vi "S4GUI_003.vi"(7 "Tab ObsEng":enum32{"Obs", "CCD modes", "Guider", "Eng"}(tab)) -> ()   [LabVIEW 2018] (continued)
              disable-tunnel: [w4939 w4953] -> w4934
              frame Disabled {
                w4952 = FALSE ("Wait Until Done")
                n2436 = call-dynamic "Read comfile name1.vi"("error in (no error)"=w4941, "Stream in"=w4944) -> ("error out"=w4940:errorcluster, "comfile name1"=w4947:string, "Stream out"=w4942:refnum<class "Stream.lvclass">)  [unwired: 7 in]
                n2437 = call <vilib>:"Application Directory.vi"() -> ("Application Directory"=w4949:path)
                n2438 = Build Path(base path=w4949, name or relative path=w4947) -> (appended path=w4948:path)
                n2439 = Open VI Reference(vi path=w4948, error in (no error)=w4940) -> (vi reference=w4950:refnum<vi>, error out=w4951:errorcluster)  [unwired: 4 in]
                n2440 = invoke class="VI" method="Run VI"(reference=w4950, error in=w4951, "Wait until done"=w4952, "Auto Dispose Ref"=w4952) -> (reference out=w4946:refnum<vi>, error out=w4945:errorcluster)  [unwired: 1 in, 3 out]
                n2441 = call-dynamic "Write commfile ref1.vi"("error in (no error)"=w4945, "commfile ref1"=w4946, "Stream in"=w4942) -> ("error out"=w4939:errorcluster, "Stream out"=w4943:refnum<class "Stream.lvclass">)  [unwired: 7 in]
              }
              frame Enabled {
              }
            }
          }
        }
        n2442 = call-dynamic "Write Stream.vi"("error in (no error)"=w4884, "Stream.lvclass"=w4885, "Server in"=w4886) -> ("error out"=w4894:errorcluster, "Server out"=w4896:refnum<class "Acquisition.lvclass">)  [unwired: 7 in]
        n2443 = call-dynamic "Write enabled.vi"("error in (no error)"=w4894, "enabled"=w4883, "Server in"=w4896) -> ("error out"=w4893:errorcluster, "Server out"=w4895:refnum<class "Acquisition.lvclass">)  [unwired: 7 in]
        n2444 = call-dynamic "Write Channel.vi"("error in (no error)"=w4893, "Channel.lvclass"=w4887, "Acquisition in"=w4895) -> ("error out"=w4901:errorcluster, "Acquisition out"=w4900:refnum<class "Acquisition.lvclass">)  [unwired: 7 in]
        n2445 = call-dynamic "Write AcquisitionD.vi"("error in (no error)"=w4901, "Acquisition.lvclass"=w4900, "S4ACS_GUI in"=w4899) -> ("error out"=w4904:errorcluster, "S4ACS_GUI out"=w4905:refnum<class "S4GUI.lvclass">)  [unwired: 7 in]
      }
      event "Run WPROT": Value Change {
        n2446 = event-data() -> ("NewVal"=w4962:bool)  [unwired: 1 in]
        n2447 = case shown="True" w4962 {
          tunnel: [u32 0 ("Ciclos  WPROT") "Ciclos  WPROT"] -> w4961
          tunnel: w4958 -> [w4964 w4969]
          tunnel: [w4964 w4968] -> w4957
          tunnel: w4956 -> [w4963 w4967]
          tunnel: [w4963 w4966] -> w4955
          frame False {
          }
          frame True {
            n2448 = call-dynamic "Write Obs_state.vi"("error in (no error)"=w4967, "Obs_state"=u32 350, "S4ACS_GUI in"=w4969) -> ("error out"=w4966:errorcluster, "S4ACS_GUI out"=w4968:refnum<class "S4GUI.lvclass">)  [unwired: 7 in]
          }
        }
        n2449 = call-dynamic "Write cycles wprot.vi"("error in (no error)"=w4955, "cycles wprot"=w4961, "S4GUI in"=w4957) -> ("error out"=w4959:errorcluster, "S4GUI out"=w4960:refnum<class "S4GUI.lvclass">)  [unwired: 7 in]
      }
      event "Start SM": Value Change {
        n2450 = event-data() -> ()  [unwired: 1 in, 6 out]
        n2451 = call-dynamic "Read Obs_state.vi"("error in (no error)"=w4998, "S4ACS_GUI in"=w4999) -> ("error out"=w4985:errorcluster, "Obs_state"=w4996:u32, "S4ACS_GUI out"=w4987:refnum<class "S4GUI.lvclass">)  [unwired: 7 in]
        n2452 = call "Read Instrument.lvclass.vi"("error in (no error)"=w4985, "S4ACS_GUI in"=w4987) -> ("error out"=w4983:errorcluster, "Instrument.lvclass"=w4984:refnum<class "Instrument.lvclass">, "S4ACS_GUI out"=w4986:refnum<class "S4GUI.lvclass">)  [unwired: 7 in]
        n2453 = Not Equal?(x=w4996, y=u32 400) -> (x != y?=w4995:bool)
        n2454 = call-dynamic "Read mode.vi"("error in (no error)"=w4983, "Instrument in"=w4984) -> ("error out"=w4982:errorcluster, "mode"=w4981:bool)  [unwired: 7 in, 1 out]
        n2455 = case shown="True" w4995 {
          tunnel: w4986 -> [w5041 w5129]
          tunnel: w4982 -> [w5042 w5128]
          tunnel: [w5045 w5135] -> w4976
          tunnel: [w5044 w5136] -> w4975
          tunnel: w4992 -> [_ w5143]
          tunnel: w4991 -> [_ w5142]
          tunnel: w4990 -> [_ w5141]
          tunnel: w4989 -> [_ w5140]
          tunnel: w4988 -> [_ w5139]
          tunnel: w4981 -> [_ w5138]
          tunnel: w4980 -> [_ w5119]
          tunnel: w4979 -> [_ w5122]
          tunnel: w4978 -> [_ w5121]
          tunnel: w4977 -> [_ w5120]
          tunnel: ["RESUME SM CLICKED" ("User Event") "START SM" ("User Event")] -> w4972
          frame False {
            # "Obs_state=400 (PAUSED), envia RESUME e vai para Obs_state=500 \npara esperar envio do comando RESUME a todos os canais."
            n2456 = call-dynamic "Write Obs_state.vi"("error in (no error)"=w5042, "Obs_state"=500, "S4ACS_GUI in"=w5041) -> ("error out"=w5046:errorcluster, "S4ACS_GUI out"=w5047:refnum<class "S4GUI.lvclass">)  [unwired: 7 in]
            n2457 = call-dynamic "Read AcquisitionA.vi"("error in (no error)"=w5046, "S4ACS_GUI in"=w5047) -> ("error out"=w5033:errorcluster, "Acquisition.lvclass"=w5037:refnum<class "Acquisition.lvclass">, "S4ACS_GUI out"=w5057:refnum<class "S4GUI.lvclass">)  [unwired: 7 in]
            n2458 = call-dynamic "Read enabled.vi"("error in (no error)"=w5033, "Server in"=w5037) -> ("error out"=w5035:errorcluster, "enabled"=w5034:bool, "Server out"=w5036:refnum<class "Acquisition.lvclass">)  [unwired: 7 in]
            n2459 = call-dynamic "Read Channel.vi"("error in (no error)"=w5035, "Acquisition in"=w5036) -> ("error out"=w5038:errorcluster, "Channel.lvclass"=w5039:refnum<class "Channel.lvclass">, "Acquisition out"=w5056:refnum<class "Acquisition.lvclass">)  [unwired: 7 in]
            n2460 = case shown="True" w5034 {
              tunnel: w5056 -> [w5104 w5117]
              tunnel: [w5104 w5116] -> w5055
              tunnel: [w5103 w5113] -> w5054
              tunnel: w5039 -> [_ w5106]
              tunnel: w5038 -> [w5103 w5105]
              frame False {
              }
              frame True {
                n2461 = call-dynamic "Read State Machine.vi"("error in (no error)"=w5105, "Device in"=w5106) -> ("error out"=w5107:errorcluster, "State Machine.lvclass"=w5108:refnum<class "State Machine.lvclass">, "Device out"=w5112:refnum<class "Channel.lvclass">)  [unwired: 7 in]
                n2462 = call "Next State.vi"("error in (no error)"=w5107, "New_State"=96, "State Machine in"=w5108) -> ("error out"=w5109:errorcluster, "State Machine out"=w5111:refnum<class "State Machine.lvclass">)  [unwired: 7 in]
                n2463 = call-dynamic "Write State Machine.vi"("error in (no error)"=w5109, "State Machine.lvclass"=w5111, "Device in"=w5112) -> ("error out"=w5114:errorcluster, "Device out"=w5115:refnum<class "Channel.lvclass">)  [unwired: 7 in]
                n2464 = call-dynamic "Write Channel.vi"("error in (no error)"=w5114, "Channel.lvclass"=w5115, "Acquisition in"=w5117) -> ("error out"=w5113:errorcluster, "Acquisition out"=w5116:refnum<class "Acquisition.lvclass">)  [unwired: 7 in]
              }
            }
            n2465 = call-dynamic "Write AcquisitionA.vi"("error in (no error)"=w5054, "Acquisition.lvclass"=w5055, "S4ACS_GUI in"=w5057) -> ("error out"=w5053:errorcluster, "S4ACS_GUI out"=w5050:refnum<class "S4GUI.lvclass">)  [unwired: 7 in]
            n2466 = call "Read AcquisitionB.vi"("error in (no error)"=w5053, "S4ACS_GUI in"=w5050) -> ("error out"=w5024:errorcluster, "Acquisition.lvclass"=w5025:refnum<class "Acquisition.lvclass">, "S4ACS_GUI out"=w5026:refnum<class "S4GUI.lvclass">)  [unwired: 7 in]
            n2467 = call-dynamic "Read enabled.vi"("error in (no error)"=w5024, "Server in"=w5025) -> ("error out"=w5028:errorcluster, "enabled"=w5027:bool, "Server out"=w5029:refnum<class "Acquisition.lvclass">)  [unwired: 7 in]
            n2468 = call-dynamic "Read Channel.vi"("error in (no error)"=w5028, "Acquisition in"=w5029) -> ("error out"=w5030:errorcluster, "Channel.lvclass"=w5031:refnum<class "Channel.lvclass">, "Acquisition out"=w5032:refnum<class "Acquisition.lvclass">)  [unwired: 7 in]
            n2469 = case shown="True" w5027 {
              tunnel: w5032 -> [w5089 w5102]
              tunnel: [w5089 w5101] -> w5023
              tunnel: [w5088 w5098] -> w5022
              tunnel: w5031 -> [_ w5091]
              tunnel: w5030 -> [w5088 w5090]
              frame False {
              }
              frame True {
                n2470 = call-dynamic "Read State Machine.vi"("error in (no error)"=w5090, "Device in"=w5091) -> ("error out"=w5092:errorcluster, "State Machine.lvclass"=w5093:refnum<class "State Machine.lvclass">, "Device out"=w5097:refnum<class "Channel.lvclass">)  [unwired: 7 in]
                n2471 = call "Next State.vi"("error in (no error)"=w5092, "New_State"=96, "State Machine in"=w5093) -> ("error out"=w5094:errorcluster, "State Machine out"=w5096:refnum<class "State Machine.lvclass">)  [unwired: 7 in]
                n2472 = call-dynamic "Write State Machine.vi"("error in (no error)"=w5094, "State Machine.lvclass"=w5096, "Device in"=w5097) -> ("error out"=w5099:errorcluster, "Device out"=w5100:refnum<class "Channel.lvclass">)  [unwired: 7 in]
                n2473 = call-dynamic "Write Channel.vi"("error in (no error)"=w5099, "Channel.lvclass"=w5100, "Acquisition in"=w5102) -> ("error out"=w5098:errorcluster, "Acquisition out"=w5101:refnum<class "Acquisition.lvclass">)  [unwired: 7 in]
              }
            }
            n2474 = call "Write AcquisitionB.vi"("error in (no error)"=w5022, "Acquisition.lvclass"=w5023, "S4ACS_GUI in"=w5026) -> ("error out"=w5052:errorcluster, "S4ACS_GUI out"=w5049:refnum<class "S4GUI.lvclass">)  [unwired: 7 in]
            n2475 = call-dynamic "Read AcquisitionC.vi"("error in (no error)"=w5052, "S4ACS_GUI in"=w5049) -> ("error out"=w5012:errorcluster, "Acquisition.lvclass"=w5015:refnum<class "Acquisition.lvclass">, "S4ACS_GUI out"=w5014:refnum<class "S4GUI.lvclass">)  [unwired: 7 in]
            n2476 = call-dynamic "Read enabled.vi"("error in (no error)"=w5012, "Server in"=w5015) -> ("error out"=w5017:errorcluster, "enabled"=w5016:bool, "Server out"=w5018:refnum<class "Acquisition.lvclass">)  [unwired: 7 in]
            n2477 = call-dynamic "Read Channel.vi"("error in (no error)"=w5017, "Acquisition in"=w5018) -> ("error out"=w5019:errorcluster, "Channel.lvclass"=w5020:refnum<class "Channel.lvclass">, "Acquisition out"=w5021:refnum<class "Acquisition.lvclass">)  [unwired: 7 in]
            n2478 = case shown="True" w5016 {
              tunnel: w5021 -> [w5074 w5087]
              tunnel: [w5074 w5086] -> w5013
              tunnel: [w5073 w5083] -> w5011
              tunnel: w5020 -> [_ w5076]
              tunnel: w5019 -> [w5073 w5075]
              frame False {
              }
              frame True {
                n2479 = call-dynamic "Read State Machine.vi"("error in (no error)"=w5075, "Device in"=w5076) -> ("error out"=w5077:errorcluster, "State Machine.lvclass"=w5078:refnum<class "State Machine.lvclass">, "Device out"=w5082:refnum<class "Channel.lvclass">)  [unwired: 7 in]
                n2480 = call "Next State.vi"("error in (no error)"=w5077, "New_State"=96, "State Machine in"=w5078) -> ("error out"=w5079:errorcluster, "State Machine out"=w5081:refnum<class "State Machine.lvclass">)  [unwired: 7 in]
                n2481 = call-dynamic "Write State Machine.vi"("error in (no error)"=w5079, "State Machine.lvclass"=w5081, "Device in"=w5082) -> ("error out"=w5084:errorcluster, "Device out"=w5085:refnum<class "Channel.lvclass">)  [unwired: 7 in]
                n2482 = call-dynamic "Write Channel.vi"("error in (no error)"=w5084, "Channel.lvclass"=w5085, "Acquisition in"=w5087) -> ("error out"=w5083:errorcluster, "Acquisition out"=w5086:refnum<class "Acquisition.lvclass">)  [unwired: 7 in]
              }
            }
            n2483 = call-dynamic "Write AcquisitionC.vi"("error in (no error)"=w5011, "Acquisition.lvclass"=w5013, "S4ACS_GUI in"=w5014) -> ("error out"=w5051:errorcluster, "S4ACS_GUI out"=w5048:refnum<class "S4GUI.lvclass">)  [unwired: 7 in]
            n2484 = call-dynamic "Read AcquisitionD.vi"("error in (no error)"=w5051, "S4ACS_GUI in"=w5048) -> ("error out"=w5002:errorcluster, "Acquisition.lvclass"=w5003:refnum<class "Acquisition.lvclass">, "S4ACS_GUI out"=w5004:refnum<class "S4GUI.lvclass">)  [unwired: 7 in]
            n2485 = call-dynamic "Read enabled.vi"("error in (no error)"=w5002, "Server in"=w5003) -> ("error out"=w5006:errorcluster, "enabled"=w5005:bool, "Server out"=w5007:refnum<class "Acquisition.lvclass">)  [unwired: 7 in]
            n2486 = call-dynamic "Read Channel.vi"("error in (no error)"=w5006, "Acquisition in"=w5007) -> ("error out"=w5008:errorcluster, "Channel.lvclass"=w5009:refnum<class "Channel.lvclass">, "Acquisition out"=w5010:refnum<class "Acquisition.lvclass">)  [unwired: 7 in]
            n2487 = case shown="True" w5005 {
              tunnel: w5010 -> [w5059 w5072]
              tunnel: [w5059 w5071] -> w5001
              tunnel: [w5058 w5068] -> w5000
              tunnel: w5009 -> [_ w5061]
              tunnel: w5008 -> [w5058 w5060]
              frame False {
              }
              frame True {
                n2488 = call-dynamic "Read State Machine.vi"("error in (no error)"=w5060, "Device in"=w5061) -> ("error out"=w5062:errorcluster, "State Machine.lvclass"=w5063:refnum<class "State Machine.lvclass">, "Device out"=w5067:refnum<class "Channel.lvclass">)  [unwired: 7 in]
                n2489 = call "Next State.vi"("error in (no error)"=w5062, "New_State"=96, "State Machine in"=w5063) -> ("error out"=w5064:errorcluster, "State Machine out"=w5066:refnum<class "State Machine.lvclass">)  [unwired: 7 in]
                n2490 = call-dynamic "Write State Machine.vi"("error in (no error)"=w5064, "State Machine.lvclass"=w5066, "Device in"=w5067) -> ("error out"=w5069:errorcluster, "Device out"=w5070:refnum<class "Channel.lvclass">)  [unwired: 7 in]
                n2491 = call-dynamic "Write Channel.vi"("error in (no error)"=w5069, "Channel.lvclass"=w5070, "Acquisition in"=w5072) -> ("error out"=w5068:errorcluster, "Acquisition out"=w5071:refnum<class "Acquisition.lvclass">)  [unwired: 7 in]
              }
            }
            n2492 = call-dynamic "Write AcquisitionD.vi"("error in (no error)"=w5000, "Acquisition.lvclass"=w5001, "S4ACS_GUI in"=w5004) -> ("error out"=w5044:errorcluster, "S4ACS_GUI out"=w5045:refnum<class "S4GUI.lvclass">)  [unwired: 7 in]
          }
          frame True {
            # "vide S4GUI:\nHandleObservationSync.vi"
            # "aba atual em Tab Acq Type"
            n2493 = call "Read Instrument.lvclass.vi"("error in (no error)"=w5128, "S4ACS_GUI in"=w5129) -> ("error out"=w5131:errorcluster, "Instrument.lvclass"=w5133:refnum<class "Instrument.lvclass">, "S4ACS_GUI out"=w5126:refnum<class "S4GUI.lvclass">)  [unwired: 7 in]
            n2494 = call "Read WPROT.vi"("error in (no error)"=w5131, "Instrument in"=w5133) -> ("error out"=w5130:errorcluster, "Opt_Selector.lvclass"=w5132:refnum<class "Opt_Selector.lvclass">)  [unwired: 7 in, 1 out]
            n2495 = call-dynamic "Read sequencia.vi"("error in (no error)"=w5130, "Opt_Selector in"=w5132) -> ("error out"=w5125:errorcluster, "sequencia"=w5127:u16)  [unwired: 7 in, 1 out]
            n2496 = case shown="\"FOCUS\"" w5119 {
              tunnel: [u32 271 ("Obs_state") u32 251 ("Obs_state")] -> w5146
              tunnel: w5126 -> [w5167 w5170]
              tunnel: w5125 -> [w5157 w5169]
              tunnel: [w5165 w5170] -> w5124
              tunnel: [w5156 w5169] -> w5123
              tunnel: w5122 -> [w5164 _]
              tunnel: w5121 -> [w5163 _]
              tunnel: w5120 -> [w5162 _]
              frame "FOCUS" {
                n2497 = call-dynamic "Read TelFocus.lvclass.vi"("error in (no error)"=w5157, "S4GUI in"=w5167) -> ("error out"=w5159:errorcluster, "TelFocus.lvclass"=w5161:refnum<class "TelFocus.lvclass">, "S4GUI out"=w5166:refnum<class "S4GUI.lvclass">)  [unwired: 7 in]
                n2498 = call-dynamic "LoadParam.vi"("#steps"=w5162, "error in (no error)"=w5159, "step"=w5163, "init"=w5164, "TelFocus in"=w5161) -> ("error out"=w5158:errorcluster, "TelFocus out"=w5160:refnum<class "TelFocus.lvclass">)  [unwired: 5 in]
                n2499 = call-dynamic "Write TelFocus.lvclass.vi"("error in (no error)"=w5158, "TelFocus.lvclass"=w5160, "S4GUI in"=w5166) -> ("error out"=w5156:errorcluster, "S4GUI out"=w5165:refnum<class "S4GUI.lvclass">)  [unwired: 7 in]
              }
              frame Default {
              }
            }
            n2500 = case shown="\"FOCUS\"" w5119 {
              tunnel: w5138 -> [_ w5152]
              tunnel: [u32 1 ("# Cycles") w5151] -> w5137
              tunnel: [u32 1 w5150] -> w5134
              tunnel: w5127 -> [_ w5149]
              frame "FOCUS" {
                # "Aba FOCUS: Para a sequencia de foco, sempre  #Cycles=1 e #Seqs=1"
              }
              frame Default {
                n2501 = case shown="False" w5152 {
                  tunnel: [0 w5155] -> w5150
                  tunnel: w5149 -> [_ w5154]
                  frame False {
                    # "OV 20230424: \n#SEQ agora armazena as\nposições da lâmina utilizadas.\nNa fotometria, #SEQ=0"
                    # "fotometria:"
                  }
                  frame True {
                    # "OV 20230424: \n#SEQ agora armazena as\nposições da lâmina utilizadas.\nNa polarimetria, #SEQ=WPROT.sequencia"
                    # "polarimetria:"
                    n2502 = To Unsigned Long Integer(number=w5154) -> (unsigned 32bit integer=w5155:u32)
                  }
                }
                n2503 = local read "# Cycles"() -> (w5151:u32)
              }
            }
            n2504 = call-dynamic "Write Obs_state.vi"("error in (no error)"=w5123, "Obs_state"=w5146, "S4ACS_GUI in"=w5124) -> ("error out"=w5145:errorcluster, "S4ACS_GUI out"=w5144:refnum<class "S4GUI.lvclass">)  [unwired: 7 in]
            n2505 = stacked-sequence {
              seq-local: [w5194 _ _ _] -> [_ w5266 _ _]
              seq-local: [w5193 _ _ _] -> [_ w5265 _ _]
              seq-local: [_ w5264 _ _] -> [_ _ w5317 _]
              seq-local: [_ w5263 _ _] -> [_ _ w5316 _]
              seq-local: [_ _ w5315 _] -> [_ _ _ w5368]
              seq-local: [_ _ w5314 _] -> [_ _ _ w5367]
              tunnel: w5145 -> [w5209 _ _ _]
              tunnel: w5144 -> [w5208 _ _ _]
              tunnel: [_ _ _ w5366] -> w5135
              tunnel: [_ _ _ w5365] -> w5136
              tunnel: w5143 -> [w5192 w5262 w5313 w5364]
              tunnel: w5142 -> [w5191 w5261 w5293 w5344]
              tunnel: w5141 -> [w5190 w5241 w5292 w5343]
              tunnel: w5140 -> [w5189 w5240 w5291 w5342]
              tunnel: w5139 -> [w5184 w5237 w5288 w5339]
              tunnel: w5137 -> [_ _ _ _]
              tunnel: w5134 -> [_ _ _ _]
              tunnel: w5119 -> [w5176 w5231 w5282 w5331]
              frame #0 {
                # "object"
                # "suffix"
                # "obsType"
                n2506 = local read "Exptime ch1"() -> (w5177:dbl)
                n2507 = call-dynamic "Read AcquisitionA.vi"("error in (no error)"=w5209, "S4ACS_GUI in"=w5208) -> ("error out"=w5207:errorcluster, "Acquisition.lvclass"=w5206:refnum<class "Acquisition.lvclass">, "S4ACS_GUI out"=w5197:refnum<class "S4GUI.lvclass">)  [unwired: 7 in]
                n2508 = call-dynamic "Read Channel.vi"("error in (no error)"=w5207, "Acquisition in"=w5206) -> ("error out"=w5204:errorcluster, "Channel.lvclass"=w5205:refnum<class "Channel.lvclass">, "Acquisition out"=w5196:refnum<class "Acquisition.lvclass">)  [unwired: 7 in]
                n2509 = call-dynamic "Read Interface.vi"("error in (no error)"=w5204, "Channel in"=w5205) -> ("error out"=w5215:errorcluster, "Interface.lvclass"=w5202:refnum<class "Interface.lvclass">, "Channel out"=w5203:refnum<class "Channel.lvclass">)  [unwired: 7 in]
                n2510 = call "Write Exposure Time.vi"("error in (no error)"=w5215, "Exposure Time"=w5177, "Interface in"=w5202) -> ("error out"=w5178:errorcluster, "Interface out"=w5181:refnum<class "Interface.lvclass">)  [unwired: 7 in]
                n2511 = case shown="Default" w5176 {
                  tunnel: w5181 -> [w5217 w5222]
                  tunnel: [w5217 w5221] -> w5180
                  tunnel: [w5216 w5220] -> w5179
                  tunnel: w5178 -> [w5216 w5219]
                  tunnel: w5177 -> [_ w5218]
                  frame "ZERO" {
                  }
                  frame Default {
                    n2512 = call-dynamic "Write prev ExpTime.vi"("error in (no error)"=w5219, "prev ExpTime"=w5218, "Interface in"=w5222) -> ("error out"=w5220:errorcluster, "Interface out"=w5221:refnum<class "Interface.lvclass">)  [unwired: 7 in]
                  }
                }
                n2513 = call-dynamic "Write Suffix.vi"("error in (no error)"=w5179, "Suffix"=w5192, "Interface in"=w5180) -> ("error out"=w5214:errorcluster, "Interface out"=w5201:refnum<class "Interface.lvclass">)  [unwired: 7 in]
                n2514 = call-dynamic "Write ObsType.vi"("error in (no error)"=w5214, "ObsType"=w5190, "Interface in"=w5201) -> ("error out"=w5213:errorcluster, "Interface out"=w5200:refnum<class "Interface.lvclass">)  [unwired: 7 in]
                n2515 = call-dynamic "Write Object.vi"("error in (no error)"=w5213, "Object"=w5189, "Interface in"=w5200) -> ("error out"=w5212:errorcluster, "Interface out"=w5199:refnum<class "Interface.lvclass">)  [unwired: 7 in]
                n2516 = call-dynamic "Write Comments.vi"("error in (no error)"=w5212, "Comments"=w5191, "Interface in"=w5199) -> ("error out"=w5211:errorcluster, "Interface out"=w5198:refnum<class "Interface.lvclass">)  [unwired: 7 in]
                n2517 = call-dynamic "Write DS9.vi"("error in (no error)"=w5211, "DS9"="F", "Interface in"=w5198) -> ("error out"=w5186:errorcluster, "Interface out"=w5188:refnum<class "Interface.lvclass">)  [unwired: 7 in]
                n2518 = call-dynamic "Write Observer.vi"("error in (no error)"=w5186, "Observer"=w5184, "Interface in"=w5188) -> ("error out"=w5185:errorcluster, "Interface out"=w5187:refnum<class "Interface.lvclass">)  [unwired: 7 in]
                n2519 = property on="Exposure Time ch1" class="Slide (strict)"("Scale.Maximum"=w5177, "Scale.Minimum"=0.0 ("Scale.Range:Minimum")) -> ()  [unwired: 2 in, 2 out]
                n2520 = call-dynamic "Write Interface.vi"("error in (no error)"=w5185, "Interface.lvclass"=w5187, "Channel in"=w5203) -> ("error out"=w5183:errorcluster, "Channel out"=w5182:refnum<class "Channel.lvclass">)  [unwired: 7 in]
                n2521 = call-dynamic "Write Channel.vi"("error in (no error)"=w5183, "Channel.lvclass"=w5182, "Acquisition in"=w5196) -> ("error out"=w5173:errorcluster, "Acquisition out"=w5175:refnum<class "Acquisition.lvclass">)  [unwired: 7 in]
                n2522 = call-dynamic "CalcCubeDuration.vi"("error in (no error)"=w5173, "Acquisition in"=w5175) -> ("error out"=w5172:errorcluster, "Acquisition out"=w5174:refnum<class "Acquisition.lvclass">)  [unwired: 8 in]
                n2523 = call-dynamic "Write AcquisitionA.vi"("error in (no error)"=w5172, "Acquisition.lvclass"=w5174, "S4ACS_GUI in"=w5197) -> ("error out"=w5193:errorcluster, "S4ACS_GUI out"=w5194:refnum<class "S4GUI.lvclass">)  [unwired: 7 in]
              }
              frame #1 {
                # "object"
                # "suffix"
                # "obsType"
                n2524 = call "Read AcquisitionB.vi"("error in (no error)"=w5265, "S4ACS_GUI in"=w5266) -> ("error out"=w5249:errorcluster, "Acquisition.lvclass"=w5250:refnum<class "Acquisition.lvclass">, "S4ACS_GUI out"=w5259:refnum<class "S4GUI.lvclass">)  [unwired: 7 in]
                n2525 = local read "Exptime ch2"() -> (w5232:dbl)
                n2526 = call-dynamic "Read Channel.vi"("error in (no error)"=w5249, "Acquisition in"=w5250) -> ("error out"=w5252:errorcluster, "Channel.lvclass"=w5251:refnum<class "Channel.lvclass">, "Acquisition out"=w5260:refnum<class "Acquisition.lvclass">)  [unwired: 7 in]
                n2527 = call-dynamic "Read Interface.vi"("error in (no error)"=w5252, "Channel in"=w5251) -> ("error out"=w5244:errorcluster, "Interface.lvclass"=w5254:refnum<class "Interface.lvclass">, "Channel out"=w5253:refnum<class "Channel.lvclass">)  [unwired: 7 in]
                n2528 = call "Write Exposure Time.vi"("error in (no error)"=w5244, "Exposure Time"=w5232, "Interface in"=w5254) -> ("error out"=w5233:errorcluster, "Interface out"=w5234:refnum<class "Interface.lvclass">)  [unwired: 7 in]
                n2529 = case shown="Default" w5231 {
                  tunnel: w5234 -> [w5268 w5273]
                  tunnel: [w5268 w5272] -> w5230
                  tunnel: [w5267 w5271] -> w5229
                  tunnel: w5233 -> [w5267 w5270]
                  tunnel: w5232 -> [_ w5269]
                  frame "ZERO" {
                  }
                  frame Default {
                    n2530 = call-dynamic "Write prev ExpTime.vi"("error in (no error)"=w5270, "prev ExpTime"=w5269, "Interface in"=w5273) -> ("error out"=w5271:errorcluster, "Interface out"=w5272:refnum<class "Interface.lvclass">)  [unwired: 7 in]
                  }
                }
                n2531 = call-dynamic "Write Suffix.vi"("error in (no error)"=w5229, "Suffix"=w5262, "Interface in"=w5230) -> ("error out"=w5245:errorcluster, "Interface out"=w5255:refnum<class "Interface.lvclass">)  [unwired: 7 in]
                n2532 = call-dynamic "Write ObsType.vi"("error in (no error)"=w5245, "ObsType"=w5241, "Interface in"=w5255) -> ("error out"=w5246:errorcluster, "Interface out"=w5256:refnum<class "Interface.lvclass">)  [unwired: 7 in]
                n2533 = call-dynamic "Write Object.vi"("error in (no error)"=w5246, "Object"=w5240, "Interface in"=w5256) -> ("error out"=w5247:errorcluster, "Interface out"=w5257:refnum<class "Interface.lvclass">)  [unwired: 7 in]
                n2534 = call-dynamic "Write Comments.vi"("error in (no error)"=w5247, "Comments"=w5261, "Interface in"=w5257) -> ("error out"=w5248:errorcluster, "Interface out"=w5258:refnum<class "Interface.lvclass">)  [unwired: 7 in]
                n2535 = call-dynamic "Write DS9.vi"("error in (no error)"=w5248, "DS9"="F", "Interface in"=w5258) -> ("error out"=w5238:errorcluster, "Interface out"=w5239:refnum<class "Interface.lvclass">)  [unwired: 7 in]
                n2536 = call-dynamic "Write Observer.vi"("error in (no error)"=w5238, "Observer"=w5237, "Interface in"=w5239) -> ("error out"=w5223:errorcluster, "Interface out"=w5224:refnum<class "Interface.lvclass">)  [unwired: 7 in]
                n2537 = property on="Exposure Time ch2" class="Slide (strict)"("Scale.Maximum"=w5232, "Scale.Minimum"=0.0 ("Scale.Range:Minimum")) -> ()  [unwired: 2 in, 2 out]
                n2538 = call-dynamic "Write Interface.vi"("error in (no error)"=w5223, "Interface.lvclass"=w5224, "Channel in"=w5253) -> ("error out"=w5236:errorcluster, "Channel out"=w5235:refnum<class "Channel.lvclass">)  [unwired: 7 in]
                n2539 = call-dynamic "Write Channel.vi"("error in (no error)"=w5236, "Channel.lvclass"=w5235, "Acquisition in"=w5260) -> ("error out"=w5226:errorcluster, "Acquisition out"=w5228:refnum<class "Acquisition.lvclass">)  [unwired: 7 in]
                n2540 = call-dynamic "CalcCubeDuration.vi"("error in (no error)"=w5226, "Acquisition in"=w5228) -> ("error out"=w5225:errorcluster, "Acquisition out"=w5227:refnum<class "Acquisition.lvclass">)  [unwired: 8 in]
                n2541 = call "Write AcquisitionB.vi"("error in (no error)"=w5225, "Acquisition.lvclass"=w5227, "S4ACS_GUI in"=w5259) -> ("error out"=w5263:errorcluster, "S4ACS_GUI out"=w5264:refnum<class "S4GUI.lvclass">)  [unwired: 7 in]
              }
              frame #2 {
                # "object"
                # "suffix"
                # "obsType"
                n2542 = call-dynamic "Read AcquisitionC.vi"("error in (no error)"=w5316, "S4ACS_GUI in"=w5317) -> ("error out"=w5307:errorcluster, "Acquisition.lvclass"=w5306:refnum<class "Acquisition.lvclass">, "S4ACS_GUI out"=w5297:refnum<class "S4GUI.lvclass">)  [unwired: 7 in]
                n2543 = call-dynamic "Read Channel.vi"("error in (no error)"=w5307, "Acquisition in"=w5306) -> ("error out"=w5304:errorcluster, "Channel.lvclass"=w5305:refnum<class "Channel.lvclass">, "Acquisition out"=w5296:refnum<class "Acquisition.lvclass">)  [unwired: 7 in]
                n2544 = local read "Exptime ch3"() -> (w5283:dbl)
                n2545 = call-dynamic "Read Interface.vi"("error in (no error)"=w5304, "Channel in"=w5305) -> ("error out"=w5312:errorcluster, "Interface.lvclass"=w5302:refnum<class "Interface.lvclass">, "Channel out"=w5303:refnum<class "Channel.lvclass">)  [unwired: 7 in]
                n2546 = call "Write Exposure Time.vi"("error in (no error)"=w5312, "Exposure Time"=w5283, "Interface in"=w5302) -> ("error out"=w5284:errorcluster, "Interface out"=w5285:refnum<class "Interface.lvclass">)  [unwired: 7 in]
                n2547 = case shown="\"ZERO\"" w5282 {
                  tunnel: w5285 -> [w5319 w5324]
                  tunnel: [w5319 w5323] -> w5281
                  tunnel: [w5318 w5322] -> w5280
                  tunnel: w5284 -> [w5318 w5321]
                  tunnel: w5283 -> [_ w5320]
                  frame "ZERO" {
                  }
                  frame Default {
                    n2548 = call-dynamic "Write prev ExpTime.vi"("error in (no error)"=w5321, "prev ExpTime"=w5320, "Interface in"=w5324) -> ("error out"=w5322:errorcluster, "Interface out"=w5323:refnum<class "Interface.lvclass">)  [unwired: 7 in]
                  }
                }
                n2549 = call-dynamic "Write Suffix.vi"("error in (no error)"=w5280, "Suffix"=w5313, "Interface in"=w5281) -> ("error out"=w5311:errorcluster, "Interface out"=w5301:refnum<class "Interface.lvclass">)  [unwired: 7 in]
                n2550 = call-dynamic "Write ObsType.vi"("error in (no error)"=w5311, "ObsType"=w5292, "Interface in"=w5301) -> ("error out"=w5310:errorcluster, "Interface out"=w5300:refnum<class "Interface.lvclass">)  [unwired: 7 in]
                n2551 = call-dynamic "Write Object.vi"("error in (no error)"=w5310, "Object"=w5291, "Interface in"=w5300) -> ("error out"=w5309:errorcluster, "Interface out"=w5299:refnum<class "Interface.lvclass">)  [unwired: 7 in]
                n2552 = call-dynamic "Write Comments.vi"("error in (no error)"=w5309, "Comments"=w5293, "Interface in"=w5299) -> ("error out"=w5308:errorcluster, "Interface out"=w5298:refnum<class "Interface.lvclass">)  [unwired: 7 in]
                n2553 = call-dynamic "Write DS9.vi"("error in (no error)"=w5308, "DS9"="F", "Interface in"=w5298) -> ("error out"=w5289:errorcluster, "Interface out"=w5290:refnum<class "Interface.lvclass">)  [unwired: 7 in]
                n2554 = property on="Exposure Time ch3" class="Slide (strict)"("Scale.Maximum"=w5283, "Scale.Minimum"=0.0 ("Scale.Range:Minimum")) -> ()  [unwired: 2 in, 2 out]
                n2555 = call-dynamic "Write Observer.vi"("error in (no error)"=w5289, "Observer"=w5288, "Interface in"=w5290) -> ("error out"=w5274:errorcluster, "Interface out"=w5275:refnum<class "Interface.lvclass">)  [unwired: 7 in]
                n2556 = call-dynamic "Write Interface.vi"("error in (no error)"=w5274, "Interface.lvclass"=w5275, "Channel in"=w5303) -> ("error out"=w5287:errorcluster, "Channel out"=w5286:refnum<class "Channel.lvclass">)  [unwired: 7 in]
                n2557 = call-dynamic "Write Channel.vi"("error in (no error)"=w5287, "Channel.lvclass"=w5286, "Acquisition in"=w5296) -> ("error out"=w5277:errorcluster, "Acquisition out"=w5279:refnum<class "Acquisition.lvclass">)  [unwired: 7 in]
                n2558 = call-dynamic "CalcCubeDuration.vi"("error in (no error)"=w5277, "Acquisition in"=w5279) -> ("error out"=w5276:errorcluster, "Acquisition out"=w5278:refnum<class "Acquisition.lvclass">)  [unwired: 8 in]
                n2559 = call-dynamic "Write AcquisitionC.vi"("error in (no error)"=w5276, "Acquisition.lvclass"=w5278, "S4ACS_GUI in"=w5297) -> ("error out"=w5314:errorcluster, "S4ACS_GUI out"=w5315:refnum<class "S4GUI.lvclass">)  [unwired: 7 in]
              }
              frame #3 {
                # "object"
                # "suffix"
                # "obsType"
                n2560 = call-dynamic "Read AcquisitionD.vi"("error in (no error)"=w5367, "S4ACS_GUI in"=w5368) -> ("error out"=w5358:errorcluster, "Acquisition.lvclass"=w5357:refnum<class "Acquisition.lvclass">, "S4ACS_GUI out"=w5348:refnum<class "S4GUI.lvclass">)  [unwired: 7 in]
                n2561 = local read "Exptime ch4"() -> (w5332:dbl)
                n2562 = call-dynamic "Read Channel.vi"("error in (no error)"=w5358, "Acquisition in"=w5357) -> ("error out"=w5355:errorcluster, "Channel.lvclass"=w5356:refnum<class "Channel.lvclass">, "Acquisition out"=w5347:refnum<class "Acquisition.lvclass">)  [unwired: 7 in]
                n2563 = call-dynamic "Read Interface.vi"("error in (no error)"=w5355, "Channel in"=w5356) -> ("error out"=w5363:errorcluster, "Interface.lvclass"=w5353:refnum<class "Interface.lvclass">, "Channel out"=w5354:refnum<class "Channel.lvclass">)  [unwired: 7 in]
                n2564 = call "Write Exposure Time.vi"("error in (no error)"=w5363, "Exposure Time"=w5332, "Interface in"=w5353) -> ("error out"=w5334:errorcluster, "Interface out"=w5336:refnum<class "Interface.lvclass">)  [unwired: 7 in]
                n2565 = case shown="Default" w5331 {
                  tunnel: w5336 -> [w5370 w5375]
                  tunnel: [w5370 w5374] -> w5335
                  tunnel: [w5369 w5373] -> w5333
                  tunnel: w5334 -> [w5369 w5372]
                  tunnel: w5332 -> [_ w5371]
                  frame "ZERO" {
                  }
                  frame Default {
                    n2566 = call-dynamic "Write prev ExpTime.vi"("error in (no error)"=w5372, "prev ExpTime"=w5371, "Interface in"=w5375) -> ("error out"=w5373:errorcluster, "Interface out"=w5374:refnum<class "Interface.lvclass">)  [unwired: 7 in]
                  }
                }
                n2567 = call-dynamic "Write Suffix.vi"("error in (no error)"=w5333, "Suffix"=w5364, "Interface in"=w5335) -> ("error out"=w5362:errorcluster, "Interface out"=w5352:refnum<class "Interface.lvclass">)  [unwired: 7 in]
                n2568 = call-dynamic "Write ObsType.vi"("error in (no error)"=w5362, "ObsType"=w5343, "Interface in"=w5352) -> ("error out"=w5361:errorcluster, "Interface out"=w5351:refnum<class "Interface.lvclass">)  [unwired: 7 in]
                n2569 = call-dynamic "Write Object.vi"("error in (no error)"=w5361, "Object"=w5342, "Interface in"=w5351) -> ("error out"=w5360:errorcluster, "Interface out"=w5350:refnum<class "Interface.lvclass">)  [unwired: 7 in]
                n2570 = call-dynamic "Write Comments.vi"("error in (no error)"=w5360, "Comments"=w5344, "Interface in"=w5350) -> ("error out"=w5359:errorcluster, "Interface out"=w5349:refnum<class "Interface.lvclass">)  [unwired: 7 in]
                n2571 = call-dynamic "Write DS9.vi"("error in (no error)"=w5359, "DS9"="F", "Interface in"=w5349) -> ("error out"=w5340:errorcluster, "Interface out"=w5341:refnum<class "Interface.lvclass">)  [unwired: 7 in]
                n2572 = property on="Exposure Time ch4" class="Slide (strict)"("Scale.Maximum"=w5332, "Scale.Minimum"=0.0 ("Scale.Range:Minimum")) -> ()  [unwired: 2 in, 2 out]
                n2573 = call-dynamic "Write Observer.vi"("error in (no error)"=w5340, "Observer"=w5339, "Interface in"=w5341) -> ("error out"=w5325:errorcluster, "Interface out"=w5326:refnum<class "Interface.lvclass">)  [unwired: 7 in]
                n2574 = call-dynamic "Write Interface.vi"("error in (no error)"=w5325, "Interface.lvclass"=w5326, "Channel in"=w5354) -> ("error out"=w5338:errorcluster, "Channel out"=w5337:refnum<class "Channel.lvclass">)  [unwired: 7 in]
                n2575 = call-dynamic "Write Channel.vi"("error in (no error)"=w5338, "Channel.lvclass"=w5337, "Acquisition in"=w5347) -> ("error out"=w5328:errorcluster, "Acquisition out"=w5330:refnum<class "Acquisition.lvclass">)  [unwired: 7 in]
                n2576 = call-dynamic "CalcCubeDuration.vi"("error in (no error)"=w5328, "Acquisition in"=w5330) -> ("error out"=w5327:errorcluster, "Acquisition out"=w5329:refnum<class "Acquisition.lvclass">)  [unwired: 8 in]
                n2577 = call-dynamic "Write AcquisitionD.vi"("error in (no error)"=w5327, "Acquisition.lvclass"=w5329, "S4ACS_GUI in"=w5348) -> ("error out"=w5365:errorcluster, "S4ACS_GUI out"=w5366:refnum<class "S4GUI.lvclass">)  [unwired: 7 in]
              }
            }
          }
        }
        n2578 = call-dynamic "Write User Event.vi"("error in (no error)"=w4975, "User Event"=w4972, "S4GUI in"=w4976) -> ("error out"=w4974:errorcluster, "S4GUI out"=w4973:refnum<class "S4GUI.lvclass">)  [unwired: 7 in]
        n2579 = property on="Pause SM" class="Bool"(error in=w4974, "DisabledEnum"=T12."Enabled" ("Disabled")) -> (error out=w4993:errorcluster)  [unwired: 1 in, 1 out]
      }
      event "# Cycles": Value Change {
        w5440 = 0.0 ("Scale.Range:Minor Increment")
        n2580 = event-data() -> ("NewVal"=w5376:u32)  [unwired: 1 in]
        n2581 = call-dynamic "Write ciclos.vi"("error in (no error)"=w5397, "ciclos"=w5376, "S4ACS_GUI in"=w5441) -> ("error out"=w5394:errorcluster, "S4ACS_GUI out"=w5396:refnum<class "S4GUI.lvclass">)  [unwired: 7 in]
        n2582 = call-dynamic "Write prev ciclos.vi"("error in (no error)"=w5394, "prev ciclos"=w5376, "S4GUI in"=w5396) -> ("error out"=w5393:errorcluster, "S4GUI out"=w5395:refnum<class "S4GUI.lvclass">)  [unwired: 7 in]
        n2583 = property on="#Cycles Done" class="Slide (strict)"("Scale.Maximum"=w5376, "Scale.Minimum"=w5440) -> ()  [unwired: 2 in, 2 out]
        n2584 = property on="Cycles Done ch2" class="Slide (strict)"("Scale.Maximum"=w5376, "Scale.Minimum"=w5440) -> ()  [unwired: 2 in, 2 out]
        n2585 = property on="Cycles Done ch4" class="Slide (strict)"("Scale.Maximum"=w5376, "Scale.Minimum"=w5440) -> ()  [unwired: 2 in, 2 out]
        n2586 = property on="Cycles Done ch1" class="Slide (strict)"("Scale.Maximum"=w5376, "Scale.Minimum"=w5440) -> ()  [unwired: 2 in, 2 out]
        n2587 = property on="Cycles Done ch3" class="Slide (strict)"("Scale.Maximum"=w5376, "Scale.Minimum"=w5440) -> ()  [unwired: 2 in, 2 out]
        n2588 = call-dynamic "Write TotalCiclos.vi"("error in (no error)"=w5393, "TotalCiclos"=w5376, "S4GUI in"=w5395) -> ("error out"=w5398:errorcluster, "S4GUI out"=w5399:refnum<class "S4GUI.lvclass">)  [unwired: 7 in]
        n2589 = call-dynamic "Read AcquisitionA.vi"("error in (no error)"=w5398, "S4ACS_GUI in"=w5399) -> ("error out"=w5434:errorcluster, "Acquisition.lvclass"=w5438:refnum<class "Acquisition.lvclass">, "S4ACS_GUI out"=w5439:refnum<class "S4GUI.lvclass">)  [unwired: 7 in]
        n2590 = call-dynamic "Read Channel.vi"("error in (no error)"=w5434, "Acquisition in"=w5438) -> ("error out"=w5433:errorcluster, "Channel.lvclass"=w5435:refnum<class "Channel.lvclass">, "Acquisition out"=w5437:refnum<class "Acquisition.lvclass">)  [unwired: 7 in]
        n2591 = call-dynamic "Write ciclos.vi"("error in (no error)"=w5433, "ciclos"=w5376, "Channel in"=w5435) -> ("error out"=w5391:errorcluster, "Channel out"=w5392:refnum<class "Channel.lvclass">)  [unwired: 7 in]
        n2592 = call-dynamic "Write prev ciclos.vi"("error in (no error)"=w5391, "prev ciclos"=w5376, "Channel in"=w5392) -> ("error out"=w5390:errorcluster, "Channel out"=w5389:refnum<class "Channel.lvclass">)  [unwired: 7 in]
        n2593 = call-dynamic "Write Channel.vi"("error in (no error)"=w5390, "Channel.lvclass"=w5389, "Acquisition in"=w5437) -> ("error out"=w5432:errorcluster, "Acquisition out"=w5436:refnum<class "Acquisition.lvclass">)  [unwired: 7 in]
        n2594 = call-dynamic "Write AcquisitionA.vi"("error in (no error)"=w5432, "Acquisition.lvclass"=w5436, "S4ACS_GUI in"=w5439) -> ("error out"=w5424:errorcluster, "S4ACS_GUI out"=w5429:refnum<class "S4GUI.lvclass">)  [unwired: 7 in]
        n2595 = call "Read AcquisitionB.vi"("error in (no error)"=w5424, "S4ACS_GUI in"=w5429) -> ("error out"=w5423:errorcluster, "Acquisition.lvclass"=w5427:refnum<class "Acquisition.lvclass">, "S4ACS_GUI out"=w5428:refnum<class "S4GUI.lvclass">)  [unwired: 7 in]
        n2596 = call-dynamic "Read Channel.vi"("error in (no error)"=w5423, "Acquisition in"=w5427) -> ("error out"=w5430:errorcluster, "Channel.lvclass"=w5431:refnum<class "Channel.lvclass">, "Acquisition out"=w5426:refnum<class "Acquisition.lvclass">)  [unwired: 7 in]
        n2597 = call-dynamic "Write ciclos.vi"("error in (no error)"=w5430, "ciclos"=w5376, "Channel in"=w5431) -> ("error out"=w5388:errorcluster, "Channel out"=w5387:refnum<class "Channel.lvclass">)  [unwired: 7 in]
        n2598 = call-dynamic "Write prev ciclos.vi"("error in (no error)"=w5388, "prev ciclos"=w5376, "Channel in"=w5387) -> ("error out"=w5385:errorcluster, "Channel out"=w5386:refnum<class "Channel.lvclass">)  [unwired: 7 in]
        n2599 = call-dynamic "Write Channel.vi"("error in (no error)"=w5385, "Channel.lvclass"=w5386, "Acquisition in"=w5426) -> ("error out"=w5422:errorcluster, "Acquisition out"=w5425:refnum<class "Acquisition.lvclass">)  [unwired: 7 in]
        n2600 = call "Write AcquisitionB.vi"("error in (no error)"=w5422, "Acquisition.lvclass"=w5425, "S4ACS_GUI in"=w5428) -> ("error out"=w5417:errorcluster, "S4ACS_GUI out"=w5418:refnum<class "S4GUI.lvclass">)  [unwired: 7 in]
        n2601 = call-dynamic "Read AcquisitionC.vi"("error in (no error)"=w5417, "S4ACS_GUI in"=w5418) -> ("error out"=w5414:errorcluster, "Acquisition.lvclass"=w5415:refnum<class "Acquisition.lvclass">, "S4ACS_GUI out"=w5416:refnum<class "S4GUI.lvclass">)  [unwired: 7 in]
        n2602 = call-dynamic "Read Channel.vi"("error in (no error)"=w5414, "Acquisition in"=w5415) -> ("error out"=w5420:errorcluster, "Channel.lvclass"=w5421:refnum<class "Channel.lvclass">, "Acquisition out"=w5419:refnum<class "Acquisition.lvclass">)  [unwired: 7 in]
        n2603 = call-dynamic "Write ciclos.vi"("error in (no error)"=w5420, "ciclos"=w5376, "Channel in"=w5421) -> ("error out"=w5383:errorcluster, "Channel out"=w5384:refnum<class "Channel.lvclass">)  [unwired: 7 in]
        n2604 = call-dynamic "Write prev ciclos.vi"("error in (no error)"=w5383, "prev ciclos"=w5376, "Channel in"=w5384) -> ("error out"=w5382:errorcluster, "Channel out"=w5381:refnum<class "Channel.lvclass">)  [unwired: 7 in]
        n2605 = call-dynamic "Write Channel.vi"("error in (no error)"=w5382, "Channel.lvclass"=w5381, "Acquisition in"=w5419) -> ("error out"=w5412:errorcluster, "Acquisition out"=w5413:refnum<class "Acquisition.lvclass">)  [unwired: 7 in]
        n2606 = call-dynamic "Write AcquisitionC.vi"("error in (no error)"=w5412, "Acquisition.lvclass"=w5413, "S4ACS_GUI in"=w5416) -> ("error out"=w5406:errorcluster, "S4ACS_GUI out"=w5407:refnum<class "S4GUI.lvclass">)  [unwired: 7 in]
        n2607 = call-dynamic "Read AcquisitionD.vi"("error in (no error)"=w5406, "S4ACS_GUI in"=w5407) -> ("error out"=w5405:errorcluster, "Acquisition.lvclass"=w5404:refnum<class "Acquisition.lvclass">, "S4ACS_GUI out"=w5408:refnum<class "S4GUI.lvclass">)  [unwired: 7 in]
        n2608 = call-dynamic "Read Channel.vi"("error in (no error)"=w5405, "Acquisition in"=w5404) -> ("error out"=w5410:errorcluster, "Channel.lvclass"=w5411:refnum<class "Channel.lvclass">, "Acquisition out"=w5409:refnum<class "Acquisition.lvclass">)  [unwired: 7 in]
        n2609 = call-dynamic "Write ciclos.vi"("error in (no error)"=w5410, "ciclos"=w5376, "Channel in"=w5411) -> ("error out"=w5379:errorcluster, "Channel out"=w5380:refnum<class "Channel.lvclass">)  [unwired: 7 in]
        n2610 = call-dynamic "Write prev ciclos.vi"("error in (no error)"=w5379, "prev ciclos"=w5376, "Channel in"=w5380) -> ("error out"=w5378:errorcluster, "Channel out"=w5377:refnum<class "Channel.lvclass">)  [unwired: 7 in]
        n2611 = call-dynamic "Write Channel.vi"("error in (no error)"=w5378, "Channel.lvclass"=w5377, "Acquisition in"=w5409) -> ("error out"=w5403:errorcluster, "Acquisition out"=w5402:refnum<class "Acquisition.lvclass">)  [unwired: 7 in]
        n2612 = call-dynamic "Write AcquisitionD.vi"("error in (no error)"=w5403, "Acquisition.lvclass"=w5402, "S4ACS_GUI in"=w5408) -> ("error out"=w5400:errorcluster, "S4ACS_GUI out"=w5401:refnum<class "S4GUI.lvclass">)  [unwired: 7 in]
      }
      event "AllConfig": Value Change {
        n2613 = event-data() -> ()  [unwired: 1 in, 6 out]
        n2614 = call "Read Instrument.lvclass.vi"("error in (no error)"=w5446, "S4ACS_GUI in"=w5447) -> ("error out"=w5526:errorcluster, "Instrument.lvclass"=w5493:refnum<class "Instrument.lvclass">, "S4ACS_GUI out"=w5524:refnum<class "S4GUI.lvclass">)  [unwired: 7 in]
        n2615 = call "Read ASEL.vi"("error in (no error)"=w5526, "Instrument in"=w5493) -> ("error out"=w5518:errorcluster, "Opt_Selector.lvclass"=w5517:refnum<class "Opt_Selector.lvclass">, "Instrument out"=w5525:refnum<class "Instrument.lvclass">)  [unwired: 7 in]
        n2616 = call-dynamic "Read State Machine.vi"("error in (no error)"=w5518, "Device in"=w5517) -> ("error out"=w5521:errorcluster, "State Machine.lvclass"=w5523:refnum<class "State Machine.lvclass">, "Device out"=w5515:refnum<class "Opt_Selector.lvclass">)  [unwired: 7 in]
        n2617 = call "Next State.vi"("error in (no error)"=w5521, "New_State"=1, "State Machine in"=w5523) -> ("error out"=w5520:errorcluster, "State Machine out"=w5519:refnum<class "State Machine.lvclass">)  [unwired: 7 in]
        n2618 = call-dynamic "Write State Machine.vi"("error in (no error)"=w5520, "State Machine.lvclass"=w5519, "Device in"=w5515) -> ("error out"=w5514:errorcluster, "Device out"=w5516:refnum<class "Opt_Selector.lvclass">)  [unwired: 7 in]
        n2619 = call "Write ASEL.vi"("error in (no error)"=w5514, "Opt_Selector.lvclass"=w5516, "Instrument in"=w5525) -> ("error out"=w5476:errorcluster, "Instrument out"=w5492:refnum<class "Instrument.lvclass">)  [unwired: 7 in]
        n2620 = call "Read CALW.vi"("error in (no error)"=w5476, "Instrument in"=w5492) -> ("error out"=w5509:errorcluster, "Opt_Selector.lvclass"=w5510:refnum<class "Opt_Selector.lvclass">, "Instrument out"=w5491:refnum<class "Instrument.lvclass">)  [unwired: 7 in]
        n2621 = call-dynamic "Read State Machine.vi"("error in (no error)"=w5509, "Device in"=w5510) -> ("error out"=w5506:errorcluster, "State Machine.lvclass"=w5504:refnum<class "State Machine.lvclass">, "Device out"=w5512:refnum<class "Opt_Selector.lvclass">)  [unwired: 7 in]
        n2622 = call "Next State.vi"("error in (no error)"=w5506, "New_State"=1, "State Machine in"=w5504) -> ("error out"=w5507:errorcluster, "State Machine out"=w5508:refnum<class "State Machine.lvclass">)  [unwired: 7 in]
        n2623 = call-dynamic "Write State Machine.vi"("error in (no error)"=w5507, "State Machine.lvclass"=w5508, "Device in"=w5512) -> ("error out"=w5513:errorcluster, "Device out"=w5511:refnum<class "Opt_Selector.lvclass">)  [unwired: 7 in]
        n2624 = call "Write CALW.vi"("error in (no error)"=w5513, "Opt_Selector.lvclass"=w5511, "Instrument in"=w5491) -> ("error out"=w5475:errorcluster, "Instrument out"=w5490:refnum<class "Instrument.lvclass">)  [unwired: 7 in]
        n2625 = call "Read WPSEL.vi"("error in (no error)"=w5475, "Instrument in"=w5490) -> ("error out"=w5498:errorcluster, "Opt_Selector.lvclass"=w5497:refnum<class "Opt_Selector.lvclass">, "Instrument out"=w5489:refnum<class "Instrument.lvclass">)  [unwired: 7 in]
        n2626 = call-dynamic "Read State Machine.vi"("error in (no error)"=w5498, "Device in"=w5497) -> ("error out"=w5501:errorcluster, "State Machine.lvclass"=w5503:refnum<class "State Machine.lvclass">, "Device out"=w5495:refnum<class "Opt_Selector.lvclass">)  [unwired: 7 in]
        n2627 = call "Next State.vi"("error in (no error)"=w5501, "New_State"=1, "State Machine in"=w5503) -> ("error out"=w5500:errorcluster, "State Machine out"=w5499:refnum<class "State Machine.lvclass">)  [unwired: 7 in]
        n2628 = call-dynamic "Write State Machine.vi"("error in (no error)"=w5500, "State Machine.lvclass"=w5499, "Device in"=w5495) -> ("error out"=w5494:errorcluster, "Device out"=w5496:refnum<class "Opt_Selector.lvclass">)  [unwired: 7 in]
        n2629 = call "Write WPSEL.vi"("error in (no error)"=w5494, "Opt_Selector.lvclass"=w5496, "Instrument in"=w5489) -> ("error out"=w5474:errorcluster, "Instrument out"=w5478:refnum<class "Instrument.lvclass">)  [unwired: 7 in]
        n2630 = call "Read WPROT.vi"("error in (no error)"=w5474, "Instrument in"=w5478) -> ("error out"=w5484:errorcluster, "Opt_Selector.lvclass"=w5485:refnum<class "Opt_Selector.lvclass">, "Instrument out"=w5477:refnum<class "Instrument.lvclass">)  [unwired: 7 in]
        n2631 = call-dynamic "Read State Machine.vi"("error in (no error)"=w5484, "Device in"=w5485) -> ("error out"=w5481:errorcluster, "State Machine.lvclass"=w5479:refnum<class "State Machine.lvclass">, "Device out"=w5487:refnum<class "Opt_Selector.lvclass">)  [unwired: 7 in]
        n2632 = call "Next State.vi"("error in (no error)"=w5481, "New_State"=1, "State Machine in"=w5479) -> ("error out"=w5482:errorcluster, "State Machine out"=w5483:refnum<class "State Machine.lvclass">)  [unwired: 7 in]
        n2633 = call-dynamic "Write State Machine.vi"("error in (no error)"=w5482, "State Machine.lvclass"=w5483, "Device in"=w5487) -> ("error out"=w5488:errorcluster, "Device out"=w5486:refnum<class "Opt_Selector.lvclass">)  [unwired: 7 in]
        n2634 = call "Write WPROT.vi"("error in (no error)"=w5488, "Opt_Selector.lvclass"=w5486, "Instrument in"=w5477) -> ("error out"=w5450:errorcluster, "Instrument out"=w5451:refnum<class "Instrument.lvclass">)  [unwired: 7 in]
        n2635 = call "Read GMIR.vi"("error in (no error)"=w5450, "Instrument in"=w5451) -> ("error out"=w5469:errorcluster, "Opt_Continuous.lvclass"=w5470:refnum<class "Opt_Continuous.lvclass">, "Instrument out"=w5463:refnum<class "Instrument.lvclass">)  [unwired: 7 in]
        n2636 = call-dynamic "Read State Machine.vi"("error in (no error)"=w5469, "Device in"=w5470) -> ("error out"=w5466:errorcluster, "State Machine.lvclass"=w5464:refnum<class "State Machine.lvclass">, "Device out"=w5472:refnum<class "Opt_Continuous.lvclass">)  [unwired: 7 in]
        n2637 = call "Next State.vi"("error in (no error)"=w5466, "New_State"=1, "State Machine in"=w5464) -> ("error out"=w5467:errorcluster, "State Machine out"=w5468:refnum<class "State Machine.lvclass">)  [unwired: 7 in]
        n2638 = call-dynamic "Write State Machine.vi"("error in (no error)"=w5467, "State Machine.lvclass"=w5468, "Device in"=w5472) -> ("error out"=w5473:errorcluster, "Device out"=w5471:refnum<class "Opt_Continuous.lvclass">)  [unwired: 7 in]
        n2639 = call "Write GMIR.vi"("error in (no error)"=w5473, "Opt_Continuous.lvclass"=w5471, "Instrument in"=w5463) -> ("error out"=w5448:errorcluster, "Instrument out"=w5449:refnum<class "Instrument.lvclass">)  [unwired: 7 in]
        n2640 = call "Read GFOC.vi"("error in (no error)"=w5448, "Instrument in"=w5449) -> ("error out"=w5458:errorcluster, "Opt_Continuous.lvclass"=w5459:refnum<class "Opt_Continuous.lvclass">, "Instrument out"=w5452:refnum<class "Instrument.lvclass">)  [unwired: 7 in]
        n2641 = call-dynamic "Read State Machine.vi"("error in (no error)"=w5458, "Device in"=w5459) -> ("error out"=w5455:errorcluster, "State Machine.lvclass"=w5453:refnum<class "State Machine.lvclass">, "Device out"=w5461:refnum<class "Opt_Continuous.lvclass">)  [unwired: 7 in]
        n2642 = call "Next State.vi"("error in (no error)"=w5455, "New_State"=1, "State Machine in"=w5453) -> ("error out"=w5456:errorcluster, "State Machine out"=w5457:refnum<class "State Machine.lvclass">)  [unwired: 7 in]
        n2643 = call-dynamic "Write State Machine.vi"("error in (no error)"=w5456, "State Machine.lvclass"=w5457, "Device in"=w5461) -> ("error out"=w5462:errorcluster, "Device out"=w5460:refnum<class "Opt_Continuous.lvclass">)  [unwired: 7 in]
